vi "Read Exception Status Response.vi"(8 "error in (no error)":errorcluster, 9 "Modbus Data Unit in":T1={"function"=1, "Data"=[]} {"function" items=["Read Discrete Inputs"=2, "Read Coils"=1, "Write Single Coil"=5, "Write Multiple Coils"=15, "Read Input Register"=4, "Read Holding Registers"=3, "Write Single Register"=6, "Write Multiple Registers"=16, "Read/Write Multiple Registers"=23, "Mask Write Register"=22, "Read FIFO Queue"=24, "Read File Record"=20, "Write File Record"=21, "Read Exception Status"=7, "Diagnostic"=8, "Get Com Event Counter"=11, "Get Com Event Log"=12, "Report Slave ID"=17, "Read Device Identification"=43]; "Data" format="%.0x"}) -> (0 "error out":errorcluster, 2 "exception status":u8)   [LabVIEW 2019, in "NI_modbus_upd.lvlib"]
doc: "Decodes the response generated by the read exception status function."
uses:
  NI_modbus_upd.lvlib
  Ctl/MB Modbus Data Unit.ctl
  Modbus Data Unit (PDU)/Function.ctl
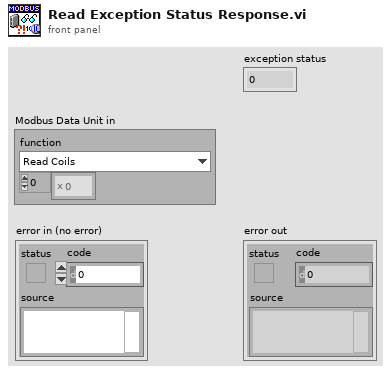
[diagram p1: front panel]
types:
  T1 = typedef "NI_modbus_upd.lvlib/MB Modbus Data Unit.ctl" = cluster{"function":T2, "Data":u8[]}
  T2 = typedef "NI_modbus_upd.lvlib/Function.ctl" = u8
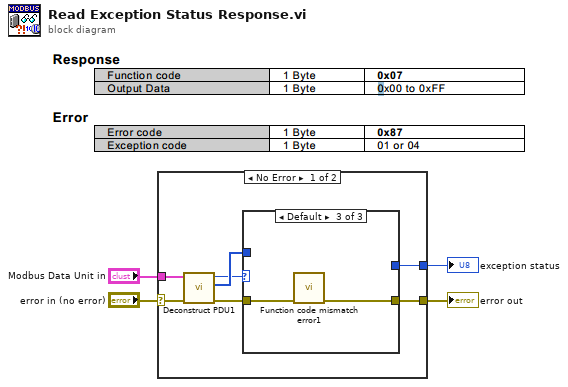
[diagram p0: block diagram]
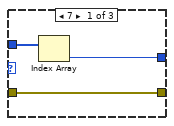
[diagram p2: hidden frame]
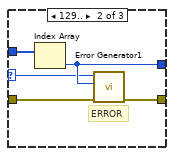
[diagram p3: hidden frame]
diagram:
  n1 = case shown="No Error" "error in (no error)" {
    selector: "error in (no error)" -> [w10 w22]
    tunnel: [w11 w22] -> w3
    tunnel: "Modbus Data Unit in" -> [w5 _]
    tunnel: [w7 _] -> w2
    frame No Error {
      n2 = call "Deconstruct PDU1.vi"("error in (no error)"=w10, "Modbus Data Unit in"=w5) -> ("error out"=w8:errorcluster, "data"=w9:u8[], "function"=w6:T2)  [unwired: 7 in]
      n3 = case shown="Default" w6 {
        selector: w6 -> [_ w15 _]
        tunnel: w8 -> [w13 w17 w21]
        tunnel: w9 -> [w14 w19 _]
        tunnel: [w13 w18 w20] -> w11
        tunnel: [w12 w16 _] -> w7
        frame 7 {
          n4 = Index Array(array=w14) -> (element=w12:u8)  [unwired: 1 in]
        }
        frame 129.. {
          # "ERROR"
          n5 = Index Array(array=w19) -> (element=w16:u8)  [unwired: 1 in]
          n6 = call "Error Generator1.vi"("error in (no error)"=w17, "data return (error code)"=w16, "function return"=w15) -> ("error out"=w18:errorcluster)  [unwired: 8 in]
        }
        frame Default {
          n7 = call "Function code mismatch error1.vi"("error in (no error)"=w21) -> ("error out"=w20:errorcluster)  [unwired: 10 in]
        }
      }
    }
    frame Error {
    }
  }
  "error out" <- w3
  "exception status" <- w2
